vi "Init Async.vi"(1 "RT Data in":T1 {"Device Channels"."Status"."BD Refs"."Data Reference" format="%.0x"; "Device Channels"."Command"."BD Refs"."Data Reference" format="%.0x"; "Local Chassis"."FPGA"."VS ref" format="%.0x"; "Local Chassis"."RSI Modules"."VS ref" format="%.0x"; "Local Chassis"."VS ref" format="%.0x"; "Device ref" format="%.0x"; "EtherCAT Masters"."REM IO ECAT Slaves"."VS ref" format="%.0x"; "EtherCAT Masters"."Generic EtherCAT Slaves"."VS ref" format="%.0x"; "EtherCAT Masters"."VS ref" format="%.0x"; "EtherCAT Masters"."EtherCAT Slaves"."FPGA"."VS ref" format="%.0x"; "EtherCAT Masters"."EtherCAT Slaves"."RSI Modules"."VS ref" format="%.0x"; "EtherCAT Masters"."EtherCAT Slaves"."VS ref" format="%.0x"}) -> (0 "RT Data out":T1 {"Device Channels"."Status"."BD Refs"."Data Reference" format="%.0x"; "Device Channels"."Command"."BD Refs"."Data Reference" format="%.0x"; "Local Chassis"."FPGA"."VS ref" format="%.0x"; "Local Chassis"."RSI Modules"."VS ref" format="%.0x"; "Local Chassis"."VS ref" format="%.0x"; "Device ref" format="%.0x"; "EtherCAT Masters"."REM IO ECAT Slaves"."VS ref" format="%.0x"; "EtherCAT Masters"."Generic EtherCAT Slaves"."VS ref" format="%.0x"; "EtherCAT Masters"."VS ref" format="%.0x"; "EtherCAT Masters"."EtherCAT Slaves"."FPGA"."VS ref" format="%.0x"; "EtherCAT Masters"."EtherCAT Slaves"."RSI Modules"."VS ref" format="%.0x"; "EtherCAT Masters"."EtherCAT Slaves"."VS ref" format="%.0x"})   [LabVIEW 2019, in "SEECD Engine.lvlib"]
uses:
  SEECD Engine.lvlib
  Type Defs/RT Data.ctl
  <vilib>/NI VeriStand/Custom Device API/Custom Device Item Ref.ctl
  Type Defs/Device Channels.ctl
  Type Defs/Output Data.ctl
  <vilib>/NI VeriStand/Custom Device API/Block Data Reference.ctl
  <vilib>/NI VeriStand/Custom Device API/Data Reference.ctl
  Type Defs/Input Data.ctl
  Type Defs/Local Chassis Data.ctl
  Type Defs/RSI Module Data.ctl
  Type Defs/Open Module IOVs.ctl
  Includes/Modules.lvlibp/RSI Module/RSI Module.lvclass
  Includes/Modules.lvlibp/RSI Module/Module Models.ctl
  Includes/Modules.lvlibp/RSI Module/Channel Type.ctl
  Type Defs/Module Config Data.ctl
  Type Defs/Mixed IO.ctl
  Type Defs/FPGA Data.ctl
  Type Defs/UDV Data.ctl
  Shared/Type Defs/UDV Data Type.ctl
  Shared/Type Defs/FXP Config.ctl
  Type Defs/Mod Size Indexes.ctl
  Type Defs/EtherCAT Master Data.ctl
  Type Defs/EtherCAT Slave Data.ctl
  Type Defs/Generic ECAT Slave RT-Data-Array.ctl
  Type Defs/Generic ECAT Slave Data Cluster.ctl
  Type Defs/Generic ECAT Slave IOV Cluster.ctl
  Type Defs/REM IO ECAT Slave RT-Data-Array.ctl
  Type Defs/REM IO ECAT Slave Data Cluster.ctl
  Type Defs/REM IO ECAT Slave IOV Cluster.ctl
  Type Defs/Async Data.ctl
  Type Defs/Async Status.ctl
  Type Defs/Async State.ctl
  Type Defs/Async Command.ctl
  Type Defs/ECAT Reconfig Data.ctl
  Type Defs/ECAT Reconfig Status.ctl
  Type Defs/ECAT Reconfig State.ctl
  Type Defs/Data Ref FGV Command.ctl
  <vilib>/NI VeriStand/Custom Device Tools/Custom Device Utility Library/Custom Device Utility Library.lvlib
  <vilib>/NI VeriStand/Custom Device API/Custom Device API.lvlib
  Shared/SEECD Shared.lvlib
types:
  T1 = typedef "SEECD Engine.lvlib/RT Data.ctl" = cluster{"Device ref":T2, "Scan Period (uSec)":u32, "Device Channels":T3, "Local Chassis":T8[], "EtherCAT Masters":T20[], "Async":T28, "ECAT Reconfig":T29, "Device Error":errorcluster, "DeviceName":string, "PCLSync?":bool}
  T2 = typedef "Custom Device API.lvlib/Custom Device Item Ref.ctl" = u64
  T3 = typedef "SEECD Engine.lvlib/Device Channels.ctl" = cluster{"Status":T4, "Command":T7}
  T4 = typedef "SEECD Engine.lvlib/Output Data.ctl" = cluster{"BD Refs":T5[], "Length":i32, "FIFO Index":i32, "Data":dbl[]}
  T5 = typedef "Custom Device API.lvlib/Block Data Reference.ctl" = cluster{"Data Reference":T6, "Offset":u64, "Length":u64}
  T6 = typedef "Custom Device API.lvlib/Data Reference.ctl" = i32
  T7 = typedef "SEECD Engine.lvlib/Input Data.ctl" = cluster{"BD Refs":T5[], "Data":dbl[], "Length":i32, "FIFO Index":i32}
  T8 = typedef "SEECD Engine.lvlib/Local Chassis Data.ctl" = cluster{"VS ref":T2, "RSI Modules":T9[], "FPGA":T15[], "Input Mod Size Idxs":T19, "Output Modules":i32[], "MixedIO Mod Size Idxs":T19}
  T9 = typedef "SEECD Engine.lvlib/RSI Module Data.ctl" = cluster{"VS ref":T2, "IOV ref":refnum<k21>, "Open Mod refs":T10, "Module DVR":refnum<data-value>, "Slot":u32, "Model":T11, "Channel Type":T12, "EtherCAT?":bool, "CDInput Data":T7, "CDOutput Data":T4, "Module Config Data":T13, "Mixed IO":T14}
  T10 = typedef "SEECD Engine.lvlib/Open Module IOVs.ctl" = cluster{"Analog Read":refnum<k21>, "Digital Read":refnum<k21>, "Analog Write":refnum<k21>, "Digital Write":refnum<k21>}
  T11 = typedef "Modules.lvlibp/RSI Module.lvclass/Module Models.ctl" = enum16{"Empty", "NI 9201", "NI 9203", "NI 9205", "NI 9206", "NI 9207", "NI 9208", "NI 9209", "NI 9210", "NI 9211", "NI 9212", "NI 9213", "NI 9214", "NI 9215", "NI 9216", "NI 9217", "NI 9219", "NI 9220", "NI 9221", "NI 9222", "NI 9223", "NI 9224", "NI 9225", "NI 9226", "NI 9227", "NI 9228", "NI 9229", "NI 9233", "NI 9234", "NI 9235", "NI 9236", "NI 9237", "NI 9239", "NI 9242", "NI 9244", "NI 9253", "NI 9263", "NI 9264", "NI 9265", "NI 9266", "NI 9269", "NI 9344", "NI 9350", "NI 9375", "NI 9401", "NI 9402", "NI 9403", "NI 9411", "NI 9421", "NI 9422", "NI 9423", "NI 9425", "NI 9426", "NI 9435", "NI 9436", "NI 9437", "NI 9472", "NI 9474", "NI 9475", "NI 9476", "NI 9477", "NI 9478", "NI 9481", "NI 9482", "NI 9485"}
  T12 = typedef "Modules.lvlibp/RSI Module.lvclass/Channel Type.ctl" = enum16{"Analog", "Digital"}
  T13 = typedef "SEECD Engine.lvlib/Module Config Data.ctl" = cluster{"Configurable?":bool, "Config Block Data Refs":T5[], "Config Data DVR":refnum<data-value>, "Previous Values":dbl[], "Local Reconfig VI Ref":refnum<vi>}
  T14 = typedef "SEECD Engine.lvlib/Mixed IO.ctl" = cluster{"Input Channel Indices":i32[], "Input Buffer":dbl[]}
  T15 = typedef "SEECD Engine.lvlib/FPGA Data.ctl" = cluster{"VS ref":T2, "IOV ref":refnum<k21>, "FPGA Target":enum16{"Local", "EtherCAT"}, "Product Code":u32, "Bitfile Signature":string, "Bitfile Path (RT)":path, "FPGA Session":u32, "Input Data":T7, "Output Data":T4, "UDVs":cluster{"From FPGA":T16[], "To FPGA":T16[]}}
  T16 = typedef "SEECD Engine.lvlib/UDV Data.ctl" = cluster{"VS ref":T2, "IOV Ref":refnum<k21>, "Name":string, "UDV Data Type":T17, "Supported Type?":bool, "FXP Config":T18, "FXP VI Ref":refnum<vi>}
  T17 = typedef "SEECD Shared.lvlib/UDV Data Type.ctl" = enum16{"Boolean", "Fixed Point", "Int8", "Int16", "Int32", "Int64", "U32 Bit Field", "UInt8", "UInt16", "UInt32", "UInt64", "Other", "DBL", "SGL"}
  T18 = typedef "SEECD Shared.lvlib/FXP Config.ctl" = cluster{"signed":bool, "size":u32, "integersize":i32}
  T19 = typedef "SEECD Engine.lvlib/Mod Size Indexes.ctl" = cluster{"4":i32[], "8":i32[], "16":i32[], "32":i32[], "other":i32[]}
  T20 = typedef "SEECD Engine.lvlib/EtherCAT Master Data.ctl" = cluster{"VS ref":T2, "IOV ref":refnum<k21>, "Master ID":u32, "Cyclic Data Bandwidth":u32, "EtherCAT Slaves":T21[], "Generic EtherCAT Slaves":T22, "REM IO ECAT Slaves":T25}
  T21 = typedef "SEECD Engine.lvlib/EtherCAT Slave Data.ctl" = cluster{"VS ref":T2, "IOV ref":refnum<k21>, "Position Address":u16, "RSI Modules":T9[], "FPGA":T15[], "Input Mod Size Idxs":T19, "Output Modules":i32[], "MixedIO Mod Size Idxs":T19}
  T22 = typedef "SEECD Engine.lvlib/Generic ECAT Slave RT-Data-Array.ctl" = T23[]
  T23 = typedef "SEECD Engine.lvlib/Generic ECAT Slave Data Cluster.ctl" = cluster{"VS ref":T2, "IOV ref":refnum<k21>, "Position Address":u16, "I/O Imput Vars ":T24[], "I/O Output Vars":T24[], "I/O Input Data":T7, "I/O Output Data":T4}
  T24 = typedef "SEECD Engine.lvlib/Generic ECAT Slave IOV Cluster.ctl" = cluster{"VS ref":T2, "IOV Ref":refnum<k21>, "Name":string, "UDV Data Type":T17}
  T25 = typedef "SEECD Engine.lvlib/REM IO ECAT Slave RT-Data-Array.ctl" = T26[]
  T26 = typedef "SEECD Engine.lvlib/REM IO ECAT Slave Data Cluster.ctl" = cluster{"VS ref":T2, "IOV ref":refnum<k21>, "Position Address":u16, "I/O Imput Vars ":T27[], "I/O Output Vars":T27[], "I/O Input Data":T7, "I/O Output Data":T4}
  T27 = typedef "SEECD Engine.lvlib/REM IO ECAT Slave IOV Cluster.ctl" = cluster{"VS ref":T2, "IOV Ref":refnum<k21>, "Name":string, "UDV Data Type":T17, "Scaling Factor":dbl}
  T28 = typedef "SEECD Engine.lvlib/Async Data.ctl" = cluster{"Status":refnum<queue>, "Command":refnum<queue>, "Input FIFO":refnum<k33>, "Input FIFO buffer":dbl[], "Output FIFO":refnum<k33>, "Output FIFO buffer":dbl[], "Async VI Ref":refnum<vi>}
  T29 = typedef "SEECD Engine.lvlib/ECAT Reconfig Data.ctl" = cluster{"Reconfig Module Found":bool, "VI Ref":refnum<vi>, "Status":refnum<queue>}
  T30 = typedef "SEECD Engine.lvlib/Async Status.ctl" = cluster{"State":T31, "error":errorcluster}
  T31 = typedef "SEECD Engine.lvlib/Async State.ctl" = enum16{"Not running", "Waiting on start cmd", "Running", "Paused", "Stopped"}
  T32 = typedef "SEECD Engine.lvlib/Async Command.ctl" = enum16{"None", "Start", "Stop"}
  T33 = typedef "SEECD Engine.lvlib/Data Ref FGV Command.ctl" = enum16{"Intialize", "Get", "Update"}
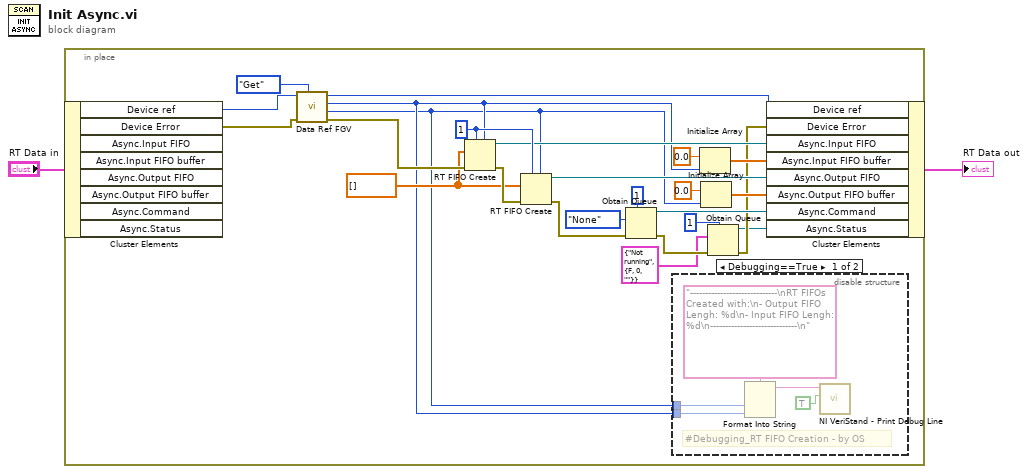
[diagram p0: block diagram]
diagram:
  n1 = in-place {
    w19 = dbl[] []
    w22 = u32 1 ("size (10)")
    n2 = in-place-cluster #1("RT Data in") -> ("Device ref"=w26:T2, "Device Error"=w25:errorcluster)  [unwired: 6 out]
    n3 = call "Data Ref FGV.vi"("Command"=Data_Ref_FGV_Command."Get", "error in (no error)"=w25, "Device Ref in"=w26) -> ("error out"=w24:errorcluster, "Output FIFO Index / Length"=w3:i32, "Input FIFO Index / Length"=w4:i32, "Device Ref out"=w21:T2)  [unwired: 5 in]
    n4 = RT FIFO Create(1:w19, 3:w24, 4:w22, 6:w4) -> (8:w20:refnum<k33>, 11:w23:errorcluster)  [unwired: 4 in, 1 out]
    n5 = RT FIFO Create(1:w19, 3:w23, 4:w22, 6:w3) -> (8:w18:refnum<k33>, 11:w10:errorcluster)  [unwired: 4 in, 1 out]
    n6 = Obtain Queue(max queue size (-1, unlimited)=1, element data type=Async_Command."None" ("Async Command"), error in (no error)=w10) -> (queue out=w11:refnum<queue>, error out=w8:errorcluster)  [unwired: 2 in, 1 out]
    n7 = disable-structure shown="Debugging==True" {
      disable-tunnel: w3 -> [w31 _]
      disable-tunnel: w4 -> [w30 _]
      frame condition #0 {
        # "#Debugging_RT FIFO Creation - by OS"
        n8 = Format Into String(format string="-----------------------------\nRT FIFOs Created with:\n- Output FIFO Lengh: %d\n- Input FIFO Lengh:    %d\n-----------------------------\n", w31, w30) -> (resulting string=w29:string)  [unwired: 2 in, 1 out]
        n9 = call <vilib>:"NI VeriStand - Print Debug Line.vi"("Add to log file? (F)"=TRUE, "Message"=w29) -> ()  [unwired: 9 in, 1 out]
      }
      frame condition #1 (active) {
      }
    }
    n10 = Initialize Array(0.0, w4) -> (w16:dbl[])
    n11 = Initialize Array(0.0, w3) -> (w14:dbl[])
    n12 = Obtain Queue(max queue size (-1, unlimited)=1, element data type=T30 {"State"=enum."Not running", "error"={"status"=FALSE, "code"=0, "source"=""}} ("Status"), error in (no error)=w8) -> (queue out=w6:refnum<queue>, error out=w9:errorcluster)  [unwired: 2 in, 1 out]
    n13 = in-place-cluster #1("Device ref"=w21, "Device Error"=w9, "Async.Input FIFO"=w20, "Async.Input FIFO buffer"=w16, "Async.Output FIFO"=w18, "Async.Output FIFO buffer"=w14, "Async.Command"=w11, "Async.Status"=w6) -> (→"RT Data out":T1)
  }
